vi "SMO.LaunchDependency.vi"(6 "Shared Resource":bool, 7 "Level":string, 8 "error in (no error)":errorcluster, 9 "Dependency Name":string, 10 "Dependency Type":refnum<class "SMO.lvclass">, 11 "SMO in":refnum<class "SMO.lvclass">) -> (0 "error out":errorcluster, 1 "Unique Name":string, 2 "Dependency Reference":refnum<class "SMO.lvclass">, 3 "SMO out":refnum<class "SMO.lvclass">)   [LabVIEW 2019, in "SMO.lvclass"]
doc: "JKI State Machine Objects (SMO) 1.3.0.56\nJKI - JKI\nCopyright (c) 2017, JKI"
uses:
  SMO.lvclass
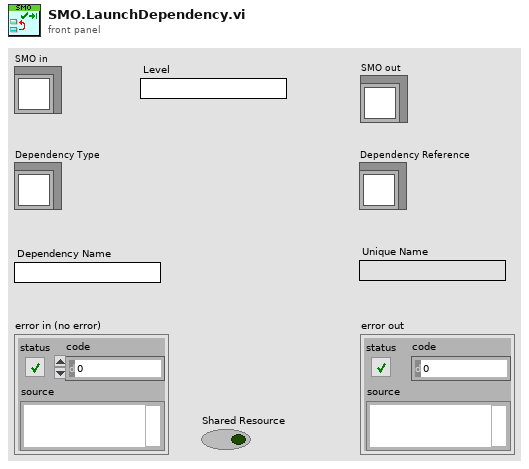
[diagram p1: front panel]
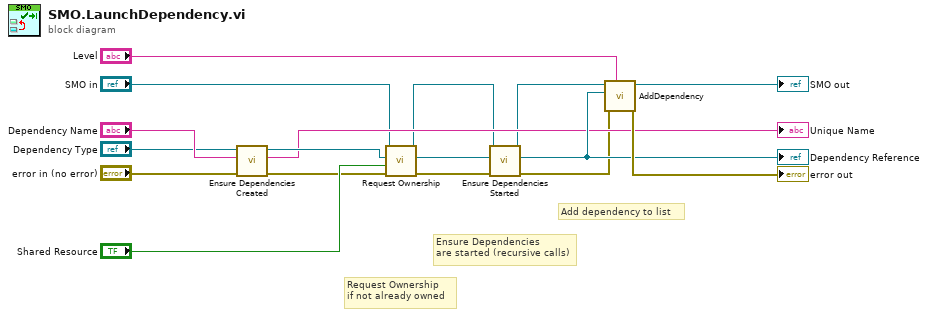
[diagram p0: block diagram]
diagram:
  # "Add dependency to list"
  # "Ensure Dependencies\nare started (recursive calls)"
  # "Request Ownership\nif not already owned"
  n1 = call "Ensure Dependencies Created.vi"("error in (no error)"="error in (no error)", "Dependency Name"="Dependency Name", "SMO in"="Dependency Type") -> ("error out"=w6:errorcluster, "Unique Dependency name"=→"Unique Name":string, "SMO out"=w15:refnum<class "SMO.lvclass">)  [unwired: 6 in]
  n2 = call "Request Ownership.vi"("error in (no error)"=w6, "Shared Resource"="Shared Resource", "Dependency"=w15, "SMO in"="SMO in") -> ("error out"=w5:errorcluster, "Dependency out"=w11:refnum<class "SMO.lvclass">, "SMO out"=w7:refnum<class "SMO.lvclass">)  [unwired: 5 in]
  n3 = call "Ensure Dependencies Started.vi"("error in (no error)"=w5, "Dependency in"=w11, "SMO in"=w7) -> ("error out"=w1:errorcluster, "Started Dependency"=w9:refnum<class "SMO.lvclass">, "SMO out"=w2:refnum<class "SMO.lvclass">)  [unwired: 6 in]
  "Dependency Reference" <- w9
  n4 = call "AddDependency.vi"("Level"="Level", "error in (no error)"=w1, "Dependency"=w9, "SMO in"=w2) -> ("error out"=→"error out":errorcluster, "SMO out"=→"SMO out":refnum<class "SMO.lvclass">)  [unwired: 6 in]
